vi "Parse Bus Controller.vi"(8 "error in (no error)":errorcluster, 11 "Bus Controller XML Node":refnum<k20>) -> (0 "error out":errorcluster, 3 "Bus Controller":refnum<class "Bus Controller.lvclass">[](array[class]))   [LabVIEW 2016]
doc: "Constructs the Bus Controller configuration and all the Frame/Message details. There can only be a single Bus Controller per Board Component. While this generates an array output, it will only ever contain a single Bus Controller."
uses:
  Bus Controller/Bus Controller.lvclass
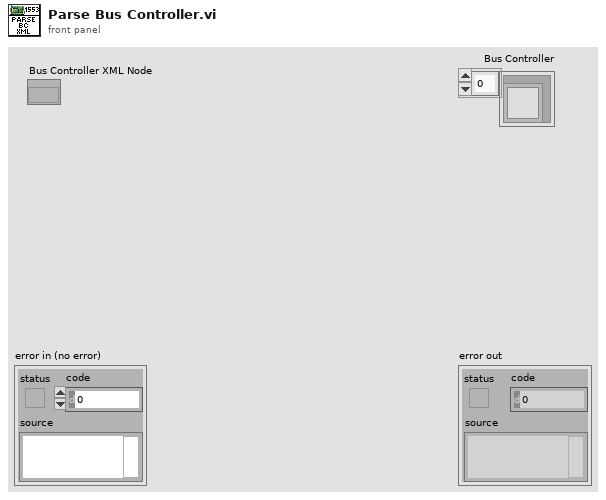
[diagram p1: front panel]
types:
  T1 = typedef "BCI-1553 API.lvlib/Bus Controller.lvclass/Bus Controller Configuration.ctl" = cluster{"BC Timeout":u16, "BC Retry":bool, "BC Second Retry":bool, "BC Retry Alt Bus":bool, "BC Second Retry Alt Bus":bool, "BC Retry on Status Bit":bool, "Msg Error No Data Valid":bool, "Busy Status No Data Valid":bool, "Msg Gap Timer":bool, "Watchdog Timer":bool, "Time Tag Sync":bool, "Even Time Tag Sync":bool, "Gap Check":bool, "Broadcast Mask Enable":bool}
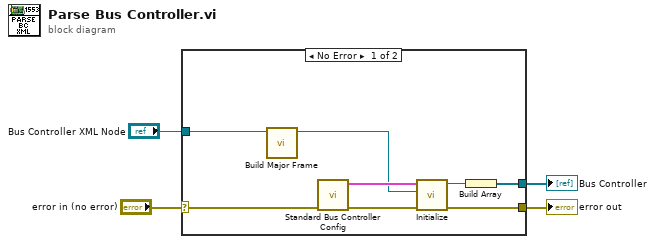
[diagram p0: block diagram]
diagram:
  n1 = case shown="No Error" "error in (no error)" {
    selector: "error in (no error)" -> [w8 w13]
    tunnel: [w11 w13] -> w3
    tunnel: [w10 _] -> w2
    tunnel: "Bus Controller XML Node" -> [w6 _]
    frame No Error {
      n2 = call "Build Major Frame.vi"("Bus Controller XML Node"=w6) -> ("Major Frame out"=w5:refnum<class "Major Frame.lvclass">)  [unwired: 9 in, 1 out]
      n3 = call "Standard Bus Controller Config.vi"("error in (no error)"=w8) -> ("error out"=w7:errorcluster, "Configuration"=w9:T1)  [unwired: 9 in]
      n4 = call "Initialize.vi"("error in (no error)"=w7, "Major Frame"=w5, "Configuration"=w9) -> ("error out"=w11:errorcluster, "Bus Controller out"=w12:refnum<class "Bus Controller.lvclass">)  [unwired: 7 in]
      n5 = Build Array(w12) -> (w10:refnum<class "Bus Controller.lvclass">[])
    }
    frame Error {
    }
  }
  "error out" <- w3
  "Bus Controller" <- w2
